vi "Vi-Sub-3-Sub-3A.vi"() -> ()   [LabVIEW 2017]
panel:
  out "Numeric":i32
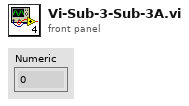
[diagram p1: front panel]
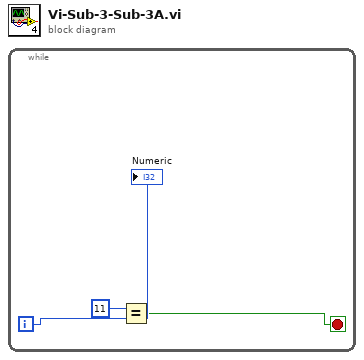
[diagram p0: block diagram]
diagram:
  n1 = while {
    i -> [w3]
    stop <- w1 stop-if-true
    n2 = Equal?(x=11, y=w3) -> (x = y?=w1:bool)
    "Numeric" <- w3
  }
